vi "Read DAQ FIFO.vi"(8 "error in (no error)":errorcluster, 9 "Timeout (ms)":i32, 10 "Data In":T1[](array[typedef]), 11 "CIF_NIChn_FIFO_DAQ in":refnum<class "CIF_NIChn_FIFO_DAQ.lvclass">) -> (0 "error out":errorcluster, 1 "timed out?":bool, 2 "Data Out":T1[](array[typedef]), 3 "CIF_NIChn_FIFO_DAQ out":refnum<class "CIF_NIChn_FIFO_DAQ.lvclass">, 4 "Header":T2)   [LabVIEW 2021, in "CIF_NIChn_FIFO_DAQ.lvclass"]
uses:
  CIF_NIChn_FIFO_DAQ.lvclass
  D:/dev/Packages/Channel_Manager/src/CIF_NIChn/FIFO_U8/CIF_NIChn_Fifo_U8.lvclass
  D:/dev/Packages/Channel_Manager/src/CIFChannels/CIFChannels.lvclass
  ChannelCommon/typedef/FIFO Header.ctl
  ChannelCommon/typedef/Datatype Waveform.ctl
  CIFChannels/CIFChannels.lvclass/CIFChannels.ctl
  NIChn/CIF_NIChn.lvclass/CIF_NIChn.ctl
  FIFO_U8/CIF_NIChn_Fifo_U8.lvclass/CIF_NIChn_Fifo_U8.ctl
  <vilib>/CIF Foundation/CIF Utilities/Statistics/I64/Stats_I64_CIF_U.lvclass/Stats_I64_CIF_U.ctl
  NIChn/Accessors/Read CIF Channel.vi
  NIChn/SubVIs/Check Disconnect.vi
  <vilib>/CIF Foundation/CIF Channels/CIFChannels/Top Level/Read U8 Array.vi
  ChannelCommon/Utilities/Unflatten Header.vi
  CIFChannels/Utilities/Update Channel Benchmark.vi
  FIFO_U8/Core/Read U8 FIFO.vi/e6dc5e5d-6043-485e-a6bf-7c23d051166d.vi
  FIFO_U8/Core/Read U8 FIFO.vi/66a3f3ff-bc1e-4ae7-83d8-3035fbf2cfec.vi
  FIFO_U8/SubVIs/Parse Payload.vi
  CIFChannels/Accessors/Read Channel State.vi
  CIFChannels/Accessors/Read Direction.vi
  SubVIs/Unflatten.vi/4ab41953-a001-49d2-beab-55370b6c3c42.vi
  SubVIs/Unflatten.vi/7cd889b7-face-4678-a9e3-2692853b6930.vi
  CIFChannels/Utilities/Update Flatten Benchmark.vi
  ChannelCommon/CIFFIFO/Flatten/Waveform Unflatten.vi
  FIFO_U8/Accessors/Read Payload.vi
  FIFO_U8/Accessors/Write Payload.vi
  CIFChannels/Accessors/Write FIFO Timeout.vi
  CIFChannels/Accessors/Write Channel State.vi
  CIFChannels/Accessors/Read Tag Disconnect Behavior.vi
  <vilib>/CIF Foundation/CIF Channels/CIFChannels/Top Level/Read U8 Array.vi/4bc1c15b-36ab-481f-b8dd-c64075ce723a.vi
  <vilib>/CIF Foundation/CIF Channels/CIFChannels/Top Level/Read U8 Array.vi/d83cb72b-7713-41fc-a3d1-682de79cf574.vi
  <vilib>/CIF Foundation/CIF Channels/CIFChannels/SubVIs/Get dll Path.vi
  <vilib>/CIF Foundation/CIF Channels/CIFChannels/SubVIs/Get Requested Size.vi
  <vilib>/CIF Foundation/CIF Utilities/DataTypes/Unflatten U64.vi
  <vilib>/CIF Foundation/CIF Utilities/DataTypes/Unflatten I64.vi
  ChannelCommon/Utilities/Add Error.vi
  <vilib>/CIF Foundation/CIF Utilities/Statistics/I64/X1 minus X0.vi
  <vilib>/CIF Foundation/CIF Utilities/Time/System Time/Get System Time.vi
  ChannelCommon/CIFFIFO/Flatten/Waveform Unflatten.vi/dd5197f3-4275-40d4-b3d5-d48df1723d2d.vi
  ChannelCommon/CIFFIFO/Flatten/Waveform Unflatten.vi/4057d038-64e5-404a-b8d2-8db20ad085cb.vi
  <vilib>/CIF Foundation/CIF Utilities/Errors/Append Error Location.vi
  <vilib>/CIF Foundation/CIF Utilities/Statistics/I64/X1 minus X0.vi/dfabcf33-0dbc-4041-80a5-3dc0c86d2989.vi
  <vilib>/CIF Foundation/CIF Utilities/Time/System Time/LabVIEW Time to TAI Time.vi
  ChannelCommon/CIFFIFO/Flatten/Waveform Unflatten.vi/dd5197f3-4275-40d4-b3d5-d48df1723d2d.vi/c28b0ead-42ad-4072-80a2-aca7f2bd7ce3.vi
  ChannelCommon/CIFFIFO/Flatten/Waveform Unflatten.vi/4057d038-64e5-404a-b8d2-8db20ad085cb.vi/c28b0ead-42ad-4072-80a2-aca7f2bd7ce3.vi
  <vilib>/CIF Foundation/CIF Utilities/Statistics/I64/X1 minus X0.vi/dfabcf33-0dbc-4041-80a5-3dc0c86d2989.vi/9eb60a9a-770f-4d2d-8b3f-8465c267ecc9.vi
  FIFO_U8/CIF_NIChn_Fifo_U8.lvclass
  D:/dev/Packages/Channel_Manager/src/CIF_NIChn/NIChn/CIF_NIChn.lvclass
  NIChn/CIF_NIChn.lvclass
  CIF_NIChn_FIFO_DAQ.lvclass/CIF_NIChn_FIFO_DAQ.ctl
  ChannelCommon/ChannelCommon.lvlib
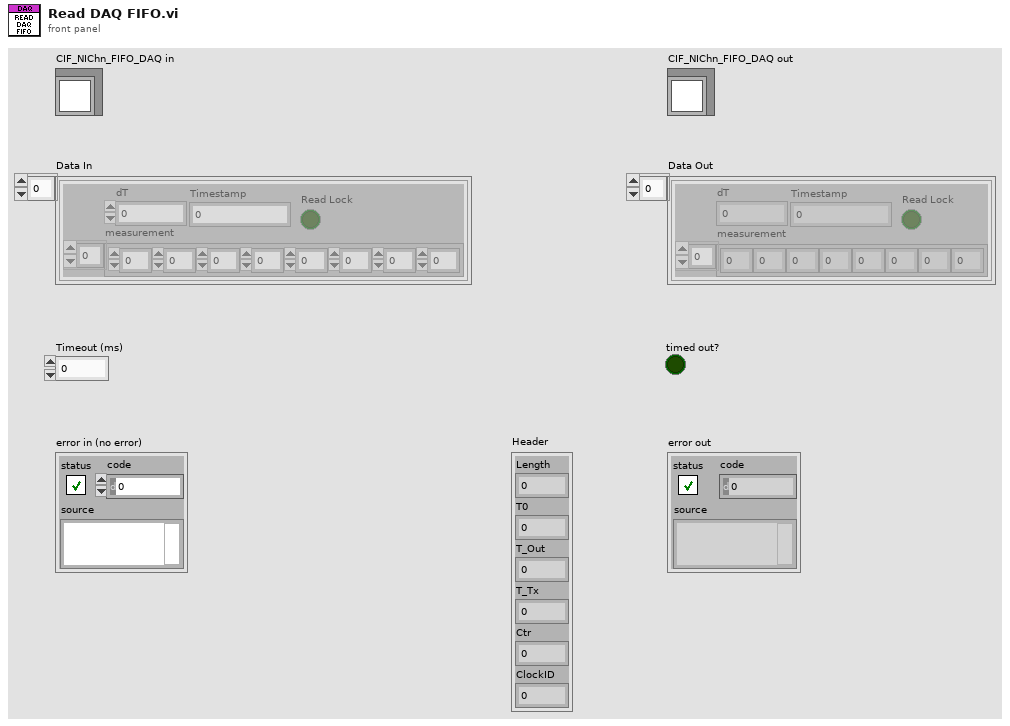
[diagram p1: front panel]
types:
  T1 = typedef "ChannelCommon.lvlib/Datatype Waveform.ctl" = cluster{"measurement":dbl[], "dT":dbl, "Timestamp":i64, "Read Lock":bool}
  T2 = typedef "ChannelCommon.lvlib/FIFO Header.ctl" = cluster{"Length":u64, "T0":i64, "T_Out":i64, "T_Tx":i64, "Ctr":u64, "ClockID":u8}
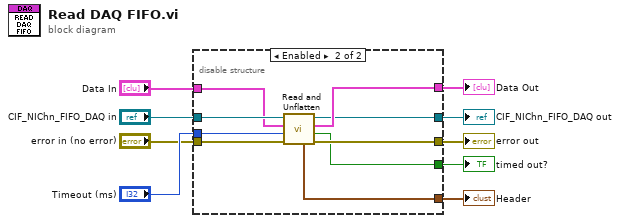
[diagram p0: block diagram]
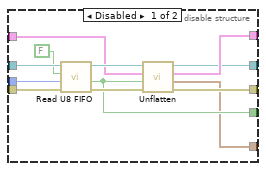
[diagram p2: hidden frame]
diagram:
  n1 = disable-structure shown="Enabled" {
    disable-tunnel: "CIF_NIChn_FIFO_DAQ in" -> [w21 w29]
    disable-tunnel: "Timeout (ms)" -> [w20 w22]
    disable-tunnel: "error in (no error)" -> [w19 w30]
    disable-tunnel: "Data In" -> [w15 w28]
    disable-tunnel: [w14 w24] -> w5
    disable-tunnel: [w13 w27] -> w4
    disable-tunnel: [w12 w26] -> w3
    disable-tunnel: [w11 w25] -> w2
    disable-tunnel: [w10 w23] -> w1
    frame Disabled {
      n2 = call "Read U8 FIFO.vi"("error in (no error)"=w19, "Timeout (ms)"=w20, "Return Data"=FALSE, "CIFFIFO in"=w21) -> ("error out"=w16:errorcluster, "timed out?"=w14:bool, "CIFFIFO out"=w18:refnum<class "CIF_NIChn_FIFO_DAQ.lvclass">)  [unwired: 3 in, 2 out]
      n3 = call "Unflatten.vi"("error in (no error)"=w16, "Timeout"=w14, "DAQ In"=w15, "CIF_NIChn_FIFO_DAQ in"=w18) -> ("error out"=w11:errorcluster, "Header"=w10:T2, "DAQ Out"=w13:T1[], "CIF_NIChn_FIFO_DAQ out"=w12:refnum<class "CIF_NIChn_FIFO_DAQ.lvclass">)  [unwired: 4 in]
    }
    frame Enabled {
      n4 = call "Read and Unflatten.vi"("error in (no error)"=w30, "Timeout (ms)"=w22, "Data in"=w28, "CIF_NIChn_FIFO_DAQ in"=w29) -> ("error out"=w25:errorcluster, "Timed out?"=w24:bool, "Data out"=w27:T1[], "CIF_NIChn_FIFO_DAQ out"=w26:refnum<class "CIF_NIChn_FIFO_DAQ.lvclass">, "Header out"=w23:T2)  [unwired: 3 in]
    }
  }
  "error out" <- w2
  "CIF_NIChn_FIFO_DAQ out" <- w3
  "timed out?" <- w5
  "Header" <- w1
  "Data Out" <- w4
